vi "CRYGet Steps From F1 F2 Resolution.vi"(8 "Steps/Tone":i32, 9 "Stop Freq":dbl, 10 "Start Freq":dbl, 11 "Resolution":u16(ring) items=["R10 (1/3 Oct.)", "R20 (1/6 Oct.)", "R40 (1/12 Oct.)", "R80 (1/24 Oct.)", "User Defined, Log", "User Defined, Linear"]) -> (1 "Stop Freq Out":dbl, 2 "Start Freq Out":dbl, 3 "Steps":i32)   [LabVIEW 2013]
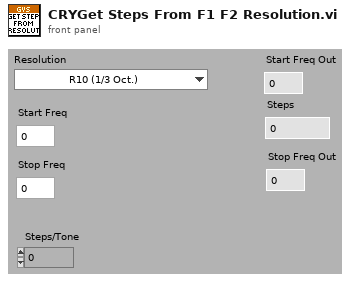
[diagram p1: front panel]
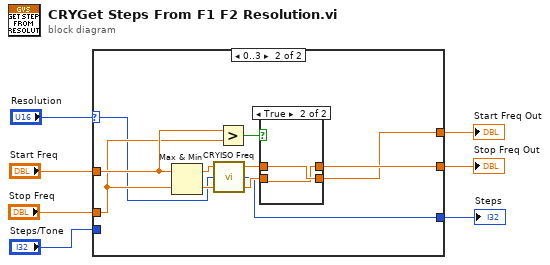
[diagram p0: block diagram]
diagram:
  n1 = case shown="0..3" "Resolution" {
    selector: "Resolution" -> [_ w11]
    tunnel: "Start Freq" -> [w10 w21]
    tunnel: "Stop Freq" -> [w9 w20]
    tunnel: [w9 w14] -> w4
    tunnel: [w10 w13] -> w3
    tunnel: [w8 w12] -> w2
    tunnel: "Steps/Tone" -> [w8 _]
    frame Default {
    }
    frame 0..3 {
      n2 = Max & Min(x=w21, y=w20) -> (max(x,y)=w16:dbl, min(x,y)=w17:dbl)
      n3 = call "CRYISO Freq.vi"("Lower Freq"=w17, "ISO series"=w11, "Higher Freq"=w16) -> ("Lower ISO Freq"=w18:dbl, "No. Steps"=w12:i32, "Higher ISO Freq"=w19:dbl)
      n4 = Greater?(x=w21, y=w20) -> (0:w15:bool)
      n5 = case shown="True" w15 {
        tunnel: [w22 w25] -> w13
        tunnel: w19 -> [w23 w25]
        tunnel: [w23 w24] -> w14
        tunnel: w18 -> [w22 w24]
        frame False {
        }
        frame True {
        }
      }
    }
  }
  "Start Freq Out" <- w3
  "Stop Freq Out" <- w4
  "Steps" <- w2
